vi "CB Test Flywheel.vi"() -> ()   [LabVIEW 2020]
uses:
  State Space/Motors/CB Motor ID.ctl
panel:
  in  "num motors":i32=1
  out "Control Effort":dbl[](graph)
  out "Reference vs State":cluster{dbl, dbl}[](graph)
  in  "moment of intertia":dbl=0.00032
  in  "gear ratio":dbl=0.66
  in  "Target":dbl(slide) scale=-1.0..1.0
  in  "r":dbl[](array[numeric])=[12.0] format="%.2f"
  in  "q":dbl[](array[numeric])=[9.42] format="%.2f"
  in  "Motor ID":T1
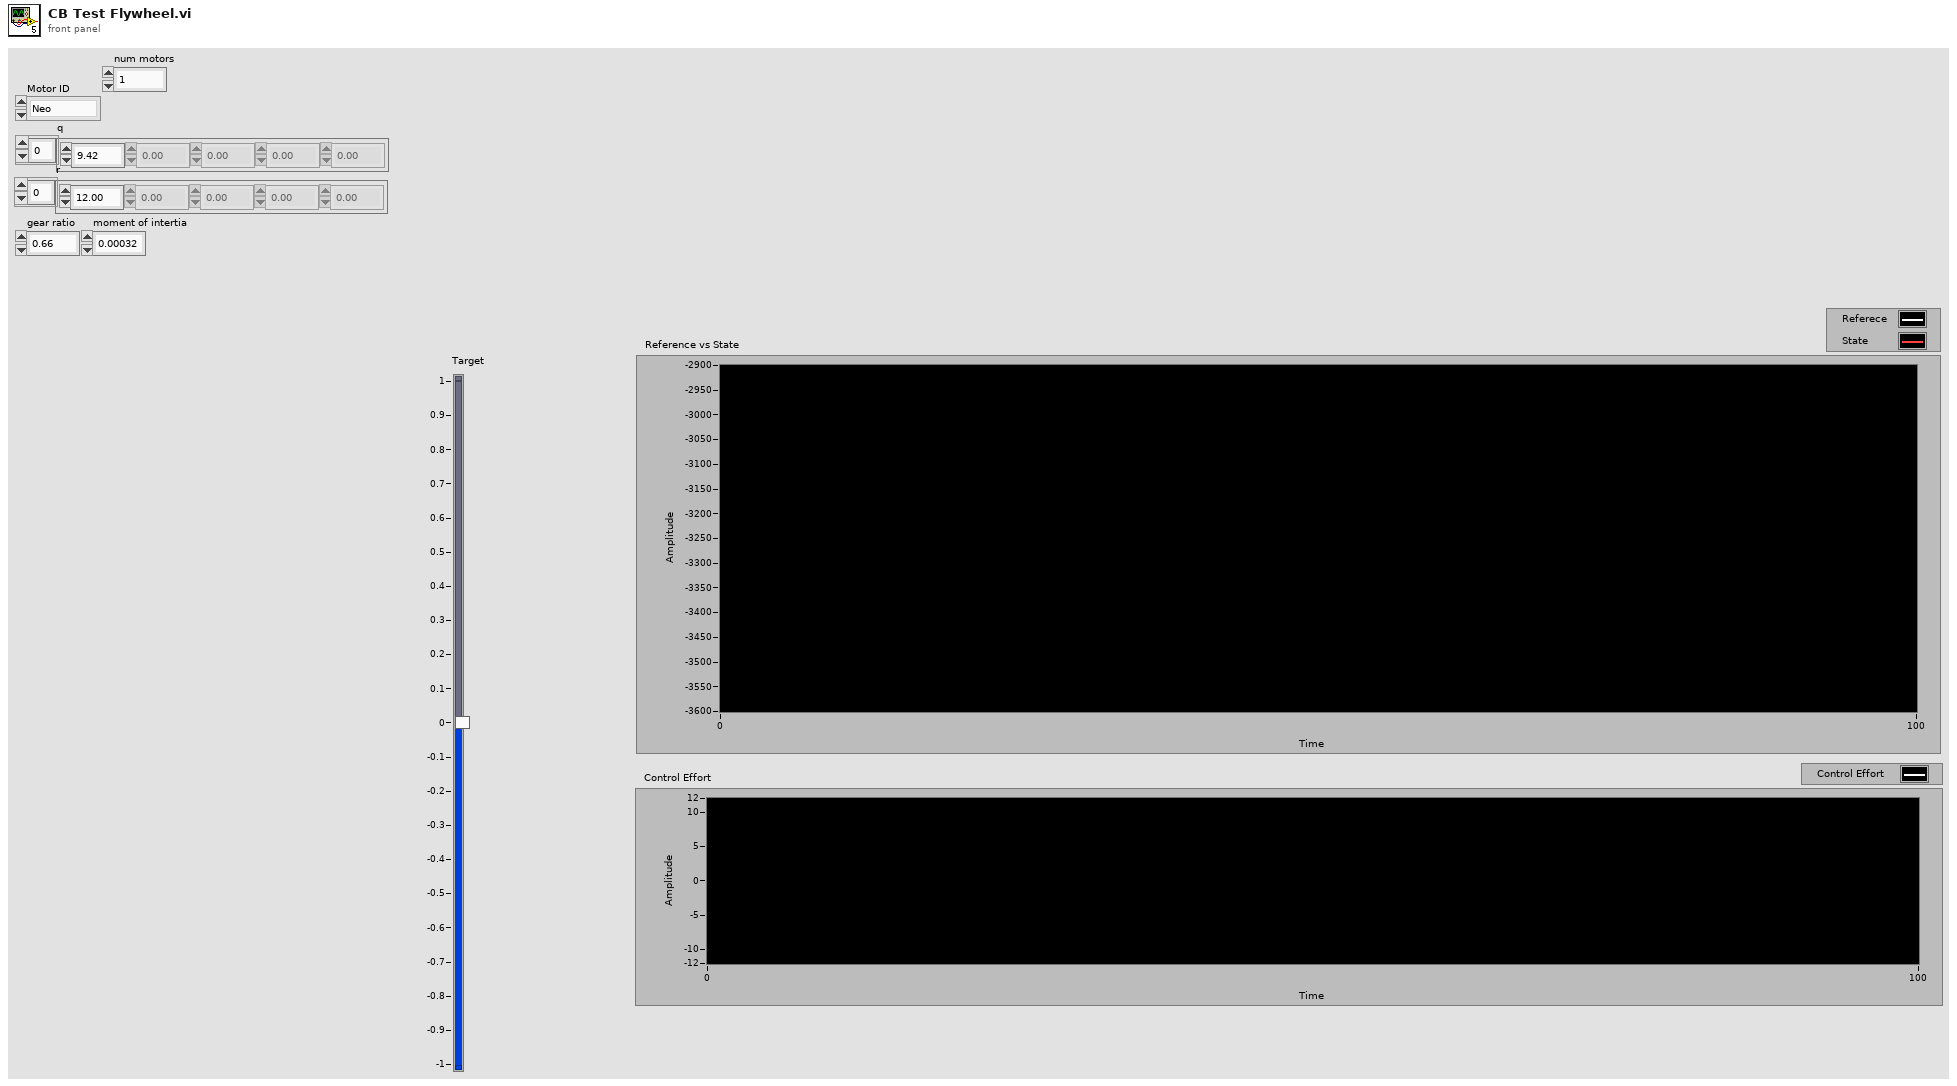
[diagram p1: front panel]
types:
  T1 = typedef "CB Motor ID.ctl" = enum16{"Neo", "Neo 550", "Falcon 500", "775pro"}
  T2 = typedef "CB State Space.ctl" = cluster{"A":T3, "B":T3, "C":T3, "D":T3, "dt":dbl}
  T3 = typedef "NI_Matrix.lvlib/RealMatrix.ctl" = dbl[][]
  T4 = cluster{"Motor ID":T1, "nominal voltage (V)":dbl, "stall torque (Nm)":dbl, "stall current (A)":dbl, "free speed (rpm)":dbl, "free current (A)":dbl}
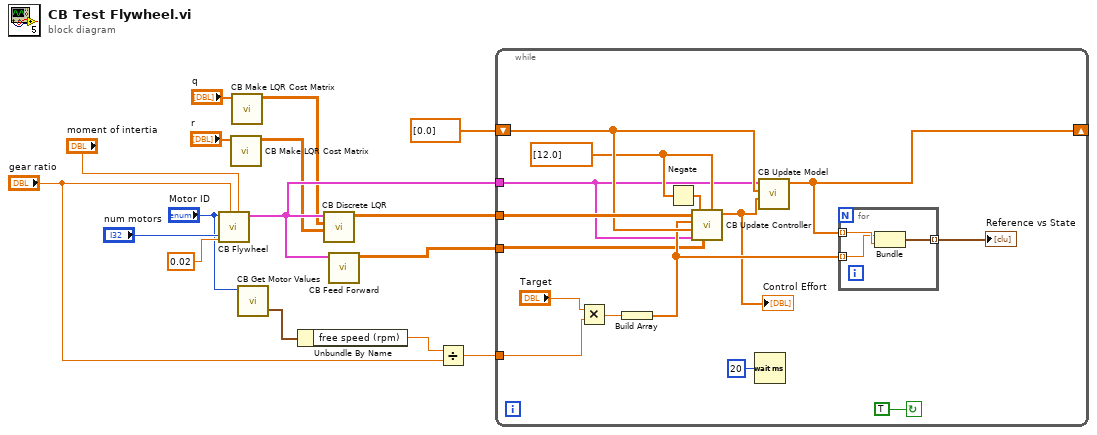
[diagram p0: block diagram]
diagram:
  n1 = call "CB Flywheel.vi"("moment of intertia"="moment of intertia", "gear ratio"="gear ratio", "dt"=0.02, "num motors"="num motors", "Motor ID"="Motor ID") -> ("Discrete SSM"=w7:T2)  [unwired: 6 in]
  n2 = call "CB Make LQR Cost Matrix.vi"("q"="r") -> ("Q"=w5:T3)  [unwired: 10 in]
  n3 = call "CB Make LQR Cost Matrix.vi"("q"="q") -> ("Q"=w6:T3)  [unwired: 10 in]
  n4 = call "CB Get Motor Values.vi"("Motor ID"="Motor ID") -> ("motor properities (single)"=w10:T4)  [unwired: 7 in, 3 out]
  n5 = Unbundle By Name(w10) -> ("free speed (rpm)"=w3:dbl)
  n6 = call "CB Discrete LQR.vi"("R"=w5, "Q"=w6, "State Space Model"=w7) -> ("K (gain matrix)"=w12:T3)  [unwired: 7 in, 1 out]
  n7 = call "CB Feed Forward.vi"("State Space Model"=w7) -> ("Feed Forward"=w4:T3)  [unwired: 10 in]
  n8 = Divide(x=w3, y="gear ratio") -> (x/y=w1:dbl)
  n9 = while {
    tunnel: w7 -> [w17]
    tunnel: w12 -> [w30]
    tunnel: w1 -> [w28]
    shift-right: [w24] -> _
    shift-left: dbl[] [0.0] ("x(k)") -> [w26]
    tunnel: w4 -> [w18]
    stop <- TRUE continue-if-true
    w20 = dbl[] [12.0] ("u_max")
    n10 = Multiply(x="Target", y=w28) -> (x*y=w27:dbl)
    n11 = Build Array(w27) -> (w23:dbl[])
    n12 = Negate(x=w20) -> (-x=w19:dbl[])
    n13 = call "CB Update Controller.vi"("u_max"=w20, "Feed Forward"=w18, "u_min"=w19, "State Space Model"=w17, "x_hat"=w26, "r(k)"=w23, "K"=w30) -> ("u"=w21:dbl[])  [unwired: 4 in]
    "Control Effort" <- w21
    n14 = Wait (ms)(milliseconds to wait=u32 20) -> ()  [unwired: 1 out]
    n15 = call "CB Update Model.vi"("u(k)"=w21, "x(k)"=w26, "State Space Model"=w17) -> ("x(k+1)"=w24:dbl[])  [unwired: 7 in, 1 out]
    n16 = for {
      tunnel: w24 -> [w34] mode=indexing
      tunnel: w23 -> [w33] mode=indexing
      tunnel: [w32] -> w22 mode=indexing
      n17 = Bundle(w33, w34) -> (w32:cluster{dbl, dbl})  [unwired: 1 in]
    }
    "Reference vs State" <- w22
  }
